vi "PQ Example SELECT, Parameters.vi"() -> ()   [LabVIEW 2015]
uses:
  Connection/Single Command (2D string).vi
  Connection/PQ Connection.lvclass
panel:
  out "Strings":string[][](array[string])
  out "error out":errorcluster
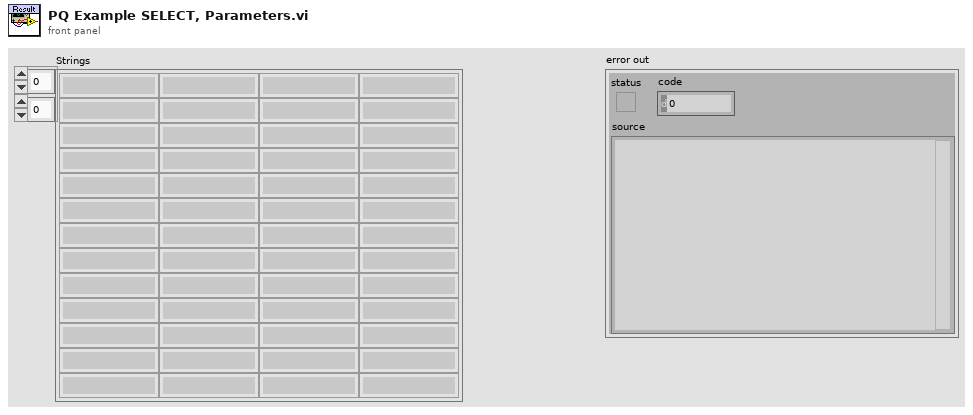
[diagram p1: front panel]
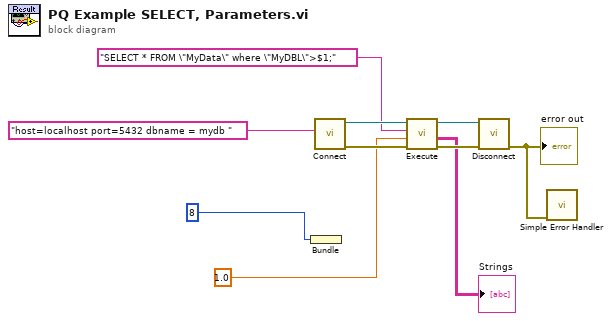
[diagram p0: block diagram]
diagram:
  n1 = Bundle(8) -> ()  [unwired: 1 in, 1 out]
  n2 = call "Connect.vi"("conninfo"="host=localhost port=5432 dbname = mydb ") -> ("error out"=w7:errorcluster, "PQ Connection out"=w9:refnum<class "PQ Connection.lvclass">)  [unwired: 9 in]
  n3 = call-poly "Execute.vi"("error in (no error)"=w7, "Variant (Cluster, Array,..)"=1.0, "SQL (Single Command)"="SELECT * FROM \"MyData\" where \"MyDBL\">$1;" ("command"), "PQ Connection in"=w9) -> ("error out"=w5:errorcluster, "Strings"=→"Strings":string[][], "PQ Connection out"=w8:refnum<class "PQ Connection.lvclass">)  [unwired: 5 in]
  n4 = call "Disconnect.vi"("error in (no error)"=w5, "PQ Connection in"=w8) -> ("error out"=w4:errorcluster)  [unwired: 9 in]
  "error out" <- w4
  n5 = call <vilib>:"Simple Error Handler.vi"("error in (no error)"=w4) -> ()  [unwired: 4 in, 5 out]
